vi "TestAuto.vi"() -> ()   [LabVIEW 2014]
panel:
  in  "stop":bool
  in  "Encoder":dbl
  in  "Manual":dbl
  in  "Button":bool
  in  "Automatic?":bool
  in  "Released?":bool=TRUE
  in  "Box Held":bool
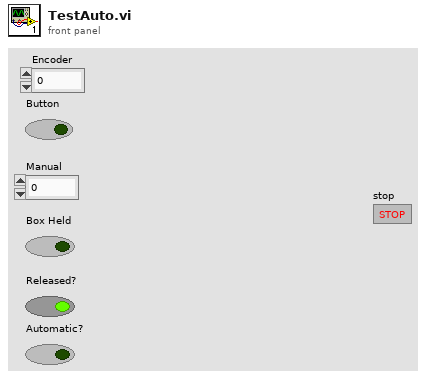
[diagram p1: front panel]
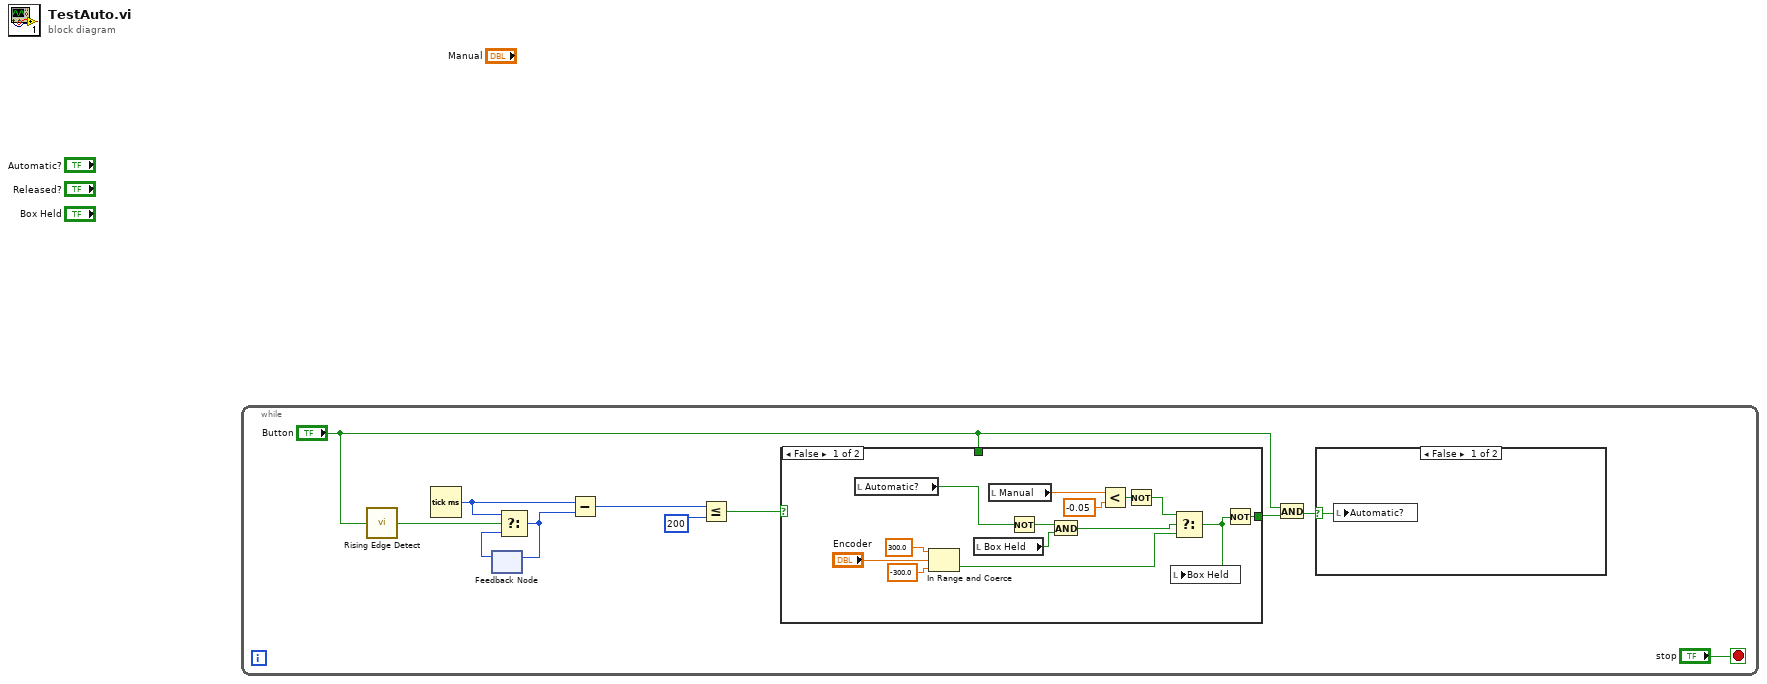
[diagram p0: block diagram]
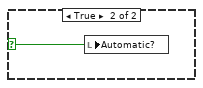
[diagram p3: hidden frame]
diagram:
  n1 = while {
    stop <- "stop" stop-if-true
    n2 = call "Rising Edge Detect.vi"("Input"="Button") -> ("Output"=w4:bool)
    n3 = Tick Count (ms)() -> (millisecond timer value=w8:u32)
    n4 = feedback #1() -> (w10:u32)  [unwired: 1 in]
    n5 = Select(t=w8, s=w4, f=w10) -> (s? t:f=w9:u32)
    n6 = feedback-in #1(w9) -> ()
    n7 = Subtract(x=w8, y=w9) -> (x-y=w7:u32)
    n8 = Less Or Equal?(x=w7, y=u32 200) -> (x <= y?=w2:bool)
    n9 = case shown="False" w2 {
      tunnel: [w19 w26] -> w3
      tunnel: "Button" -> [_ w26]
      frame False {
        n10 = local read "Automatic?"() -> (w15:bool)
        n11 = In Range and Coerce(upper limit=300.0, x="Encoder", lower limit=-300.0) -> (In Range?=w20:bool)  [unwired: 1 out]
        n12 = local read "Box Held"() -> (w13:bool)
        n13 = local read "Manual"() -> (w18:dbl)
        n14 = Not(x=w15) -> (.not. x?=w14:bool)
        n15 = And(x=w14, y=w13) -> (x .and. y?=w12:bool)
        n16 = Less?(x=w18, y=-0.05) -> (x < y?=w22:bool)
        n17 = Not(x=w22) -> (.not. x?=w16:bool)
        n18 = Select(t=w16, s=w12, f=w20) -> (s? t:f=w21:bool)
        n19 = local write "Box Held"(w21) -> ()
        n20 = Not(x=w21) -> (.not. x?=w19:bool)
      }
      frame True {
      }
    }
    n21 = And(x="Button", y=w3) -> (x .and. y?=w11:bool)
    n22 = case shown="False" w11 {
      selector: w11 -> [w27 w28]
      frame False {
        n23 = local write "Automatic?"(w27) -> ()
      }
      frame True {
        n24 = local write "Automatic?"(w28) -> ()
      }
    }
  }
